vi "Keithley 2000 Read Multiple.vi"() -> ()   [LabVIEW 2020]
doc: "This example shows how to select a function, use a trigger delay, and read multiple measurements. It also shows how to calculate the timeout for multiple measurements based on the trigger delay and the number of points."
uses:
  <instrlib>/Keithley 2000/Public/Configure/Configure DC Volts.vi
  <instrlib>/Keithley 2000/Public/Configure/Configure AC Volts.vi
  <instrlib>/Keithley 2000/Public/Configure/Configure DC Current.vi
  <instrlib>/Keithley 2000/Public/Configure/Configure AC Current.vi
  <instrlib>/Keithley 2000/Public/Configure/Configure 2 Wire Resistance.vi
  <instrlib>/Keithley 2000/Public/Configure/Configure 4 Wire Resistance.vi
  <instrlib>/Keithley 2000/Keithley 2000.lvlib
panel:
  out "Waveform Chart":dbl[](graph)
  in  "Function (0: DC Volts)":u16(ring) items=["DC Volts", "AC Volts", "DC Current", "AC Current", "2-Wire Resistance", "4-Wire Resistance"]
  in  "VISA resource name":refnum<visa-resource-name>
  out "Units":string[](array[string])
  in  "Delay (0 s)":dbl
  in  "Number of Readings (10)":i32=10
  out "Data":dbl[](array[numeric]) format="%^_8g"
  # "© 2003, National Instruments, Corporation.  All Rights Reserved."
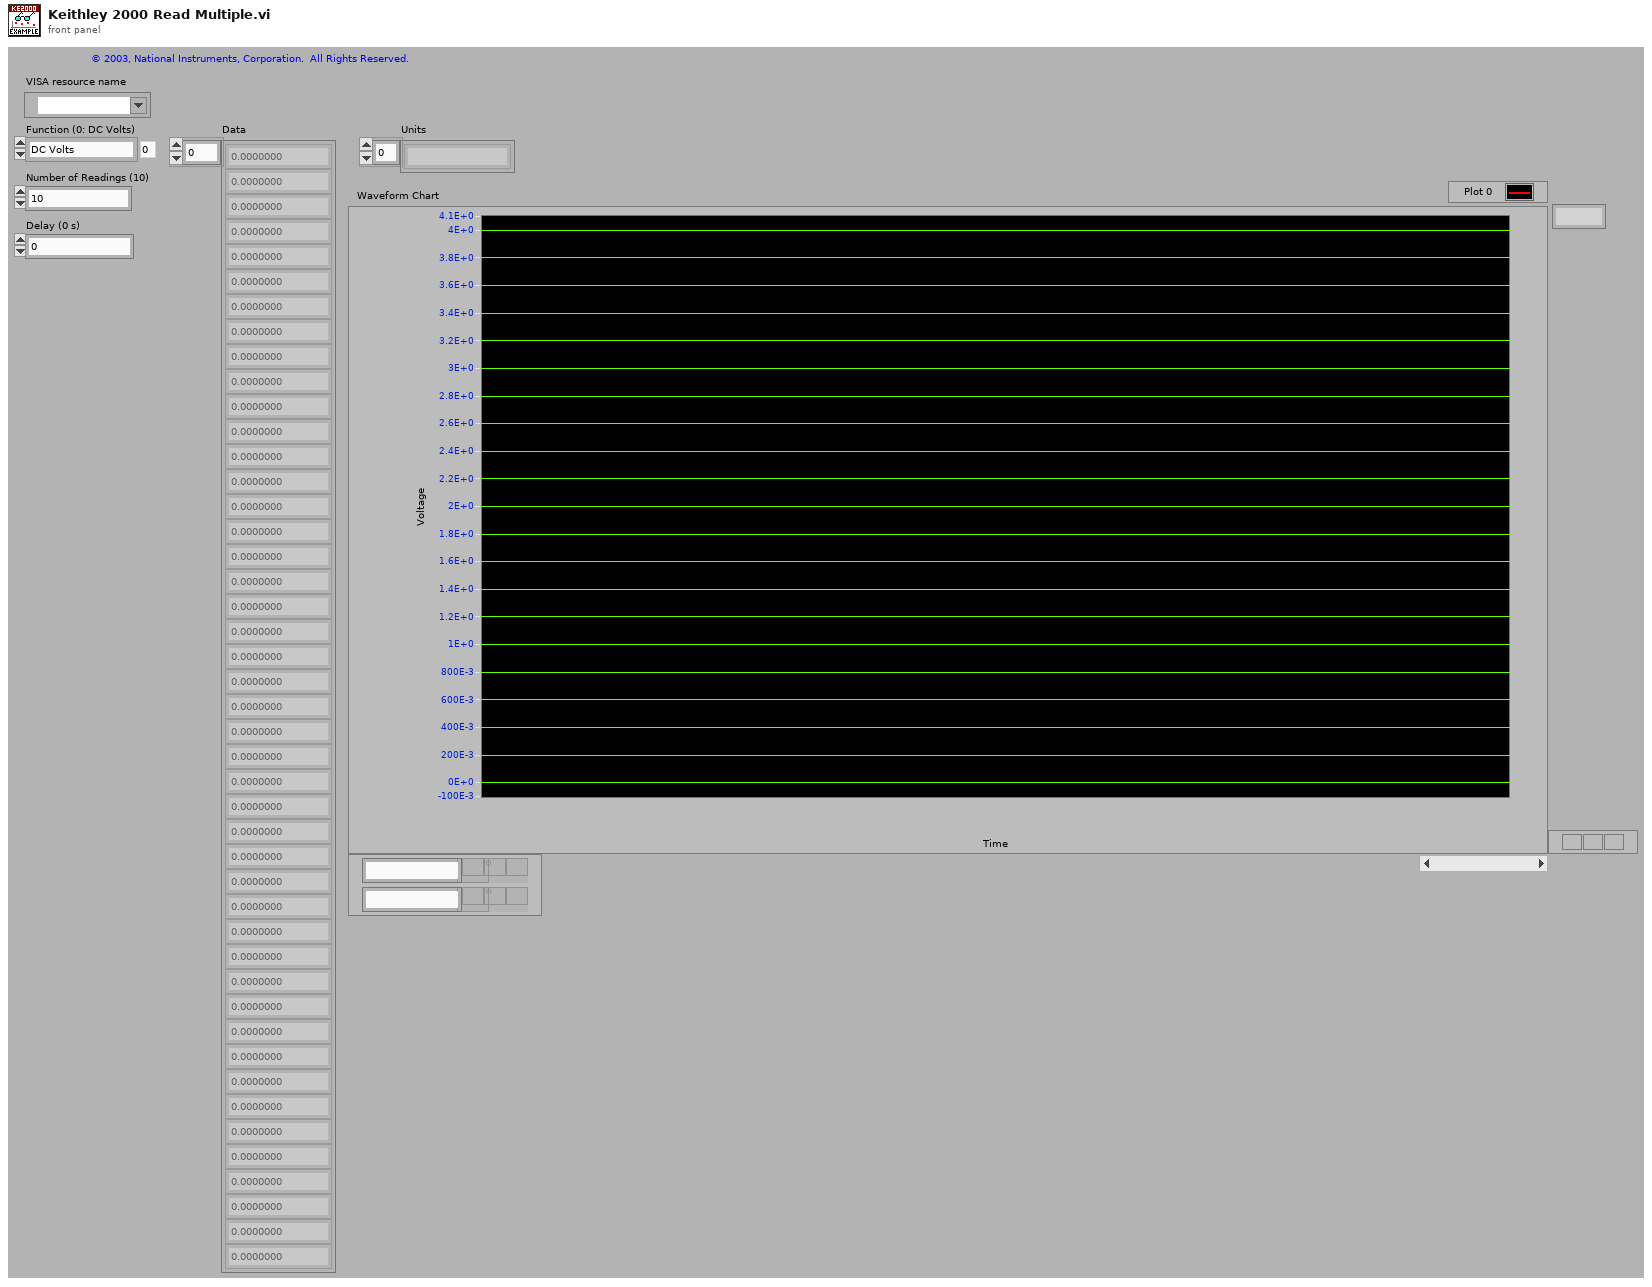
[diagram p1: front panel]
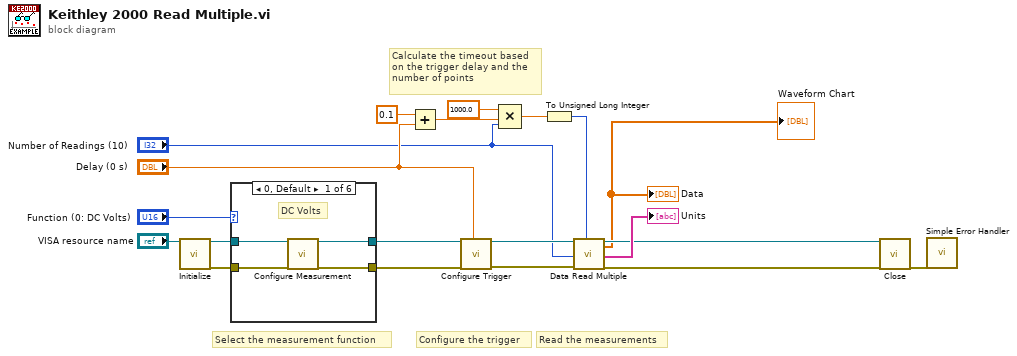
[diagram p0: block diagram]
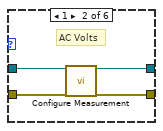
[diagram p2: hidden frame]
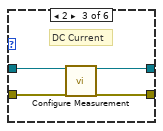
[diagram p3: hidden frame]
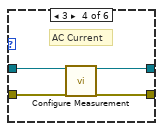
[diagram p4: hidden frame]
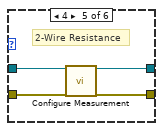
[diagram p5: hidden frame]
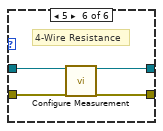
[diagram p6: hidden frame]
diagram:
  # "Read the measurements"
  # "Configure the trigger"
  # "Select the measurement function"
  # "Calculate the timeout based\non the trigger delay and the\nnumber of points"
  n1 = call <instrlib>:"Initialize.vi"("VISA resource name"="VISA resource name") -> ("VISA resource name out"=w3:refnum<visa-resource-name>, "error out"=w2:errorcluster)  [unwired: 17 in]
  n2 = case shown="0, Default" "Function (0: DC Volts)" {
    tunnel: w2 -> [w21 w28 w32 w36 w40 w44]
    tunnel: w3 -> [w24 w27 w31 w35 w39 w43]
    tunnel: [w23 w26 w30 w34 w38 w42] -> w4
    tunnel: [w22 w25 w29 w33 w37 w41] -> w5
    frame 0, Default {
      # "DC Volts"
      n3 = call-poly <instrlib>:"Configure Measurement.vi"("VISA resource name"=w24, "error in (no error)"=w21) -> ("VISA resource name out"=w22:refnum<visa-resource-name>, "error out"=w23:errorcluster)  [unwired: 16 in]
    }
    frame 1 {
      # "AC Volts"
      n4 = call-poly <instrlib>:"Configure Measurement.vi"("VISA resource name"=w27, "error in (no error)"=w28) -> ("VISA resource name out"=w25:refnum<visa-resource-name>, "error out"=w26:errorcluster)  [unwired: 16 in]
    }
    frame 2 {
      # "DC Current"
      n5 = call-poly <instrlib>:"Configure Measurement.vi"("VISA resource name"=w31, "error in (no error)"=w32) -> ("VISA resource name out"=w29:refnum<visa-resource-name>, "error out"=w30:errorcluster)  [unwired: 16 in]
    }
    frame 3 {
      # "AC Current"
      n6 = call-poly <instrlib>:"Configure Measurement.vi"("VISA resource name"=w35, "error in (no error)"=w36) -> ("VISA resource name out"=w33:refnum<visa-resource-name>, "error out"=w34:errorcluster)  [unwired: 16 in]
    }
    frame 4 {
      # "2-Wire Resistance"
      n7 = call-poly <instrlib>:"Configure Measurement.vi"("VISA resource name"=w39, "error in (no error)"=w40) -> ("VISA resource name out"=w37:refnum<visa-resource-name>, "error out"=w38:errorcluster)  [unwired: 16 in]
    }
    frame 5 {
      # "4-Wire Resistance"
      n8 = call-poly <instrlib>:"Configure Measurement.vi"("VISA resource name"=w43, "error in (no error)"=w44) -> ("VISA resource name out"=w41:refnum<visa-resource-name>, "error out"=w42:errorcluster)  [unwired: 16 in]
    }
  }
  n9 = Add(x=0.1, y="Delay (0 s)") -> (x+y=w9:dbl)
  n10 = call <instrlib>:"Configure Trigger.vi"("VISA resource name"=w5, "error in (no error)"=w4, "Delay (0 s)"="Delay (0 s)") -> ("VISA resource name out"=w16:refnum<visa-resource-name>, "error out"=w15:errorcluster)  [unwired: 15 in]
  n11 = Compound Arithmetic op=MULTIPLY(1000.0 ("x"), w9, "Number of Readings (10)") -> (w7:dbl)
  n12 = To Unsigned Long Integer(number=w7) -> (unsigned 32bit integer=w11:u32)
  n13 = call <instrlib>:"Data Read Multiple.vi"("VISA resource name"=w16, "Number of Readings (100)"="Number of Readings (10)", "error in (no error)"=w15, "Timeout (25000 ms)"=w11) -> ("VISA resource name out"=w17:refnum<visa-resource-name>, "Data"=→"Data" →"Waveform Chart":dbl[], "Units"=→"Units":string[], "error out"=w18:errorcluster)  [unwired: 11 in, 1 out]
  n14 = call <instrlib>:"Close.vi"("VISA resource name"=w17, "error in (no error)"=w18) -> ("error out"=w20:errorcluster)  [unwired: 17 in]
  n15 = call <vilib>:"Simple Error Handler.vi"("error in (no error)"=w20) -> ()  [unwired: 4 in, 5 out]
